vi "Write Differential Speed Msg.vi"(3 "Use PWM?":bool, 4 "Offset":i32=200, 5 "Right Controller Y Axis":i32, 6 "Left Controller Y Axis":i32) -> (0 "Left Motor":i16, 1 "Right Motor":i16, 2 "Speed UDP Message":string)   [LabVIEW 2015]
uses:
  <vilib>/gmath/NI_Gmath.lvlib
panel:
  out "Content length":i32
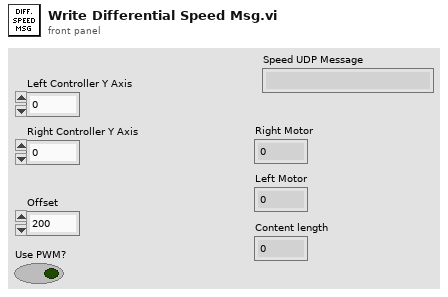
[diagram p1: front panel]
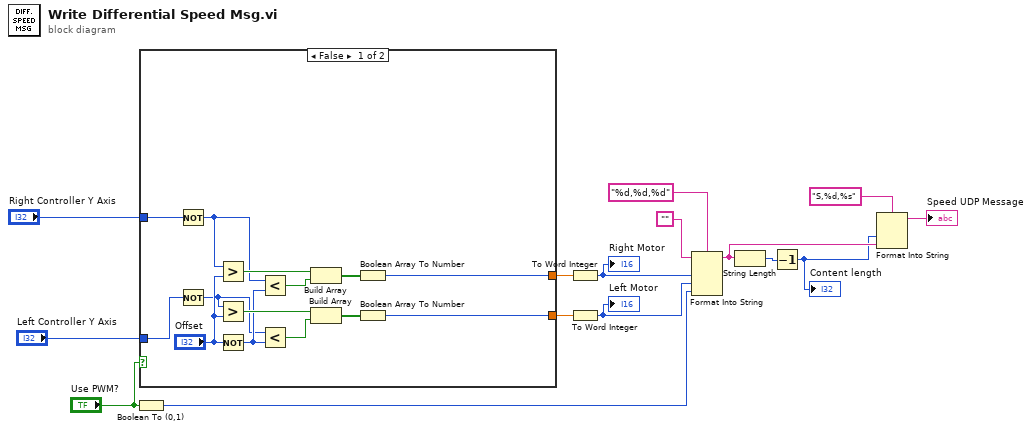
[diagram p0: block diagram]
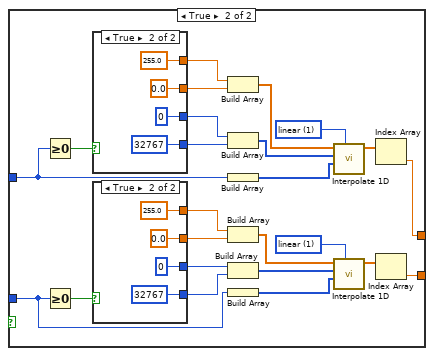
[diagram p2: hidden frame]
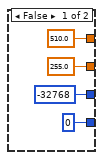
[diagram p3: hidden frame]
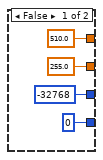
[diagram p4: hidden frame]
diagram:
  n1 = Boolean To (0,1)(Boolean="Use PWM?") -> (0, 1=w2:i16)
  n2 = case shown="False" "Use PWM?" {
    tunnel: [w21 w42] -> w10
    tunnel: [w20 w30] -> w9
    tunnel: "Right Controller Y Axis" -> [w19 w46]
    tunnel: "Left Controller Y Axis" -> [w18 w31]
    frame False {
      n3 = Not(x=w19) -> (.not. x?=w16:i32)
      n4 = Not(x=w18) -> (.not. x?=w17:i32)
      n5 = Greater?(x=w16, y="Offset") -> (0:w25:bool)
      n6 = Greater?(x=w17, y="Offset") -> (0:w29:bool)
      n7 = Not(x="Offset") -> (.not. x?=w22:i32)
      n8 = Less?(x=w16, y=w22) -> (x < y?=w26:bool)
      n9 = Less?(x=w17, y=w22) -> (x < y?=w28:bool)
      n10 = Build Array(w25, w26) -> (w24:bool[])
      n11 = Build Array(w29, w28) -> (w27:bool[])
      n12 = Boolean Array To Number(Boolean array=w24) -> (number=w21:u32)
      n13 = Boolean Array To Number(Boolean array=w27) -> (number=w20:u32)
    }
    frame True {
      w33 = 1 items=["nearest", "linear", "spline", "cubic Hermite", "Lagrange"] ("method")
      w53 = 1 items=["nearest", "linear", "spline", "cubic Hermite", "Lagrange"] ("method")
      n14 = Greater Or Equal To 0?(x=w46) -> (x >= 0?=w44:bool)
      n15 = Greater Or Equal To 0?(x=w31) -> (x >= 0?=w32:bool)
      n16 = case shown="True" w44 {
        tunnel: [i16 0 i16 32767 ("element")] -> w50
        tunnel: [i16 -32768 i16 0] -> w49
        tunnel: [255.0 ("element") 0.0 ("element")] -> w48
        tunnel: [510.0 ("element") 255.0 ("element")] -> w47
        frame False {
        }
        frame True {
        }
      }
      n17 = case shown="True" w32 {
        tunnel: [i16 0 i16 32767 ("element")] -> w36
        tunnel: [i16 -32768 i16 0] -> w37
        tunnel: [255.0 ("element") 0.0 ("element")] -> w38
        tunnel: [510.0 ("element") 255.0 ("element")] -> w39
        frame False {
        }
        frame True {
        }
      }
      n18 = Build Array(w47, w48) -> (w51:dbl[])
      n19 = Build Array(w49, w50) -> (w52:i16[])
      n20 = Build Array(w46) -> (w45:i32[])
      n21 = Build Array(w39, w38) -> (w35:dbl[])
      n22 = Build Array(w37, w36) -> (w34:i16[])
      n23 = Build Array(w31) -> (w40:i32[])
      n24 = call <vilib>:"Interpolate 1D.vi"("method"=w53, "xi"=w45, "X"=w52, "Y"=w51) -> ("yi"=w43:dbl[])  [unwired: 5 in, 2 out]
      n25 = call <vilib>:"Interpolate 1D.vi"("method"=w33, "xi"=w40, "X"=w34, "Y"=w35) -> ("yi"=w41:dbl[])  [unwired: 5 in, 2 out]
      n26 = Index Array(array=w43) -> (element=w42:dbl)  [unwired: 1 in]
      n27 = Index Array(array=w41) -> (element=w30:dbl)  [unwired: 1 in]
    }
  }
  n28 = To Word Integer(number=w10) -> (16bit integer=w8:i16)
  "Right Motor" <- w8
  n29 = To Word Integer(number=w9) -> (16bit integer=w7:i16)
  "Left Motor" <- w7
  n30 = Format Into String(format string="%d,%d,%d", initial string="", w8, w7, w2) -> (resulting string=w13:string)  [unwired: 1 in, 1 out]
  n31 = String Length(string=w13) -> (length=w4:i32)
  n32 = Decrement(x=w4) -> (x-1=w3:i32)
  "Content length" <- w3
  n33 = Format Into String(format string="S,%d,%s", w3, w13) -> (resulting string=→"Speed UDP Message":string)  [unwired: 2 in, 1 out]
